vi "Autonomous.vi"   [LabVIEW 2017]
doc: "This VI starts when autonomous period begins, and will automatically be terminated when it ends. You can carry out timed or sensor driven operations directly to I/O or to subsystems without needing to return to the caller."
uses:
  <vilib>/Rock Robotics/WPI/Utilities/WPI_GetSetVariantRefNum.vi
  <vilib>/Rock Robotics/Network Tables/NT Read String.vi
types:
  T1 = typedef "Command Status Info.ctl" = cluster{"Name":string, "Status":T2, "notifier out":T3}
  T2 = typedef "Completion Status.ctl" = enum16{"Successful", "Aborted", "Incomplete"}
  T3 = typedef "Completion Notifier.ctl" = refnum<notifier>
  T4 = typedef "WPI_JoystickDevRef.ctl" = cluster{"Device":T5}
  T5 = typedef "WPI_JoystickDeviceEnum.ctl" = enum16{"USB 0", "USB 1", "USB 2", "USB 3", "USB 4", "USB 5"}
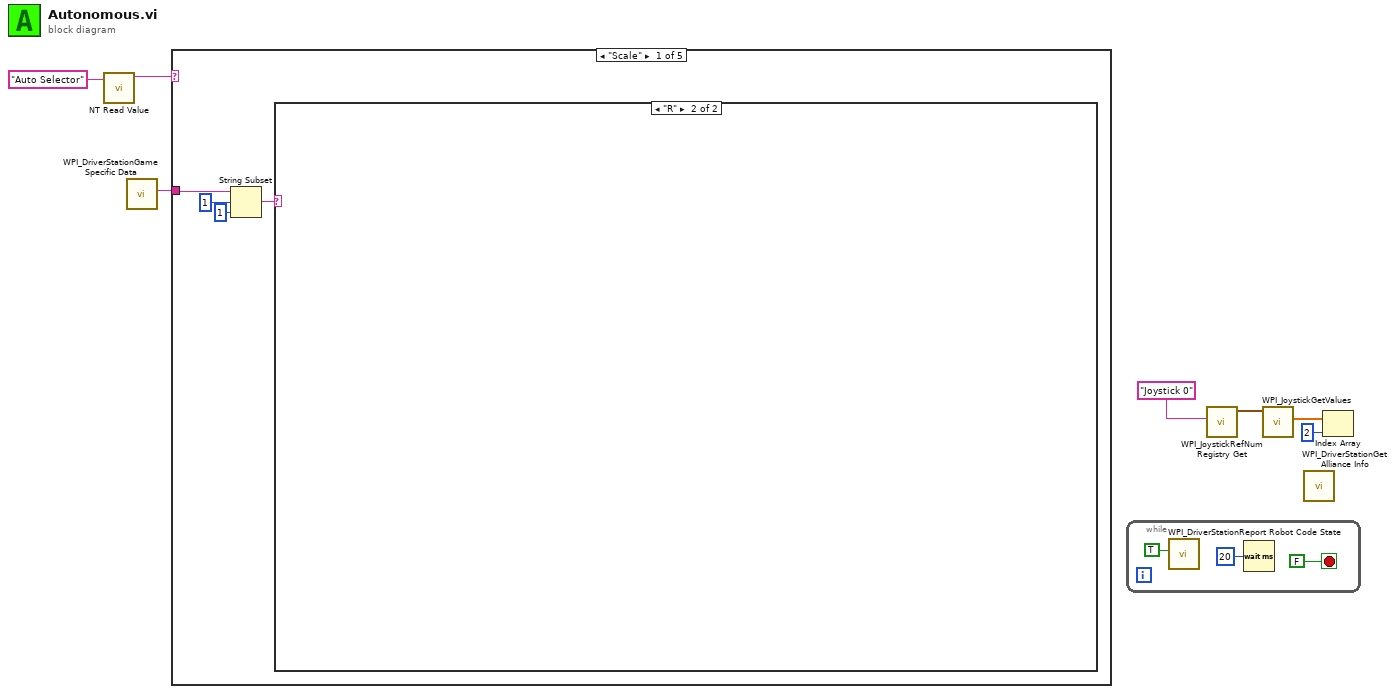
[diagram p0: block diagram]
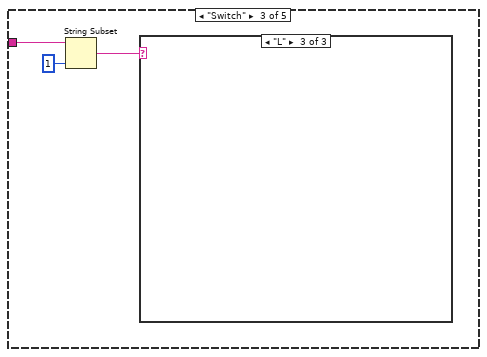
[diagram p4: hidden frame]
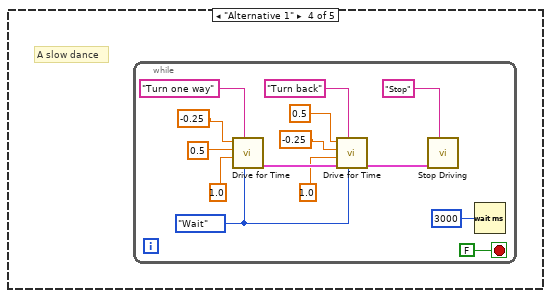
[diagram p7: hidden frame]
diagram:
  n1 = call-poly <vilib>:"NT Read Value.vi"("Name"="Auto Selector") -> ("String"=w2:string)  [unwired: 9 in, 1 out]
  n2 = call <vilib>:"WPI_DriverStationGame Specific Data.vi"() -> ("Game Specific Data"=w1:string)  [unwired: 11 in]
  n3 = case shown="\"Scale\"" w2 {
    tunnel: w1 -> [w11 _ w14 _ _]
    frame "Scale" {
      n4 = String Subset(string=w11, offset (0)=1, length (rest)=1 ("length (rest)")) -> (substring=w8:string)
      n5 = case shown="\"R\"" w8 {
        frame "L", Default {
        }
        frame "R" {
        }
      }
    }
    frame "Baseline" {
    }
    frame "Switch" {
      n6 = String Subset(string=w14, length (rest)=1 ("length (rest)")) -> (substring=w13:string)  [unwired: 1 in]
      n7 = case shown="\"L\"" w13 {
        frame "Def", Default {
        }
        frame "R" {
        }
        frame "L" {
        }
      }
    }
    frame "Alternative 1" {
      # "A slow dance"
      n8 = while {
        stop <- FALSE stop-if-true
        w19 = enum16{"Start", "Wait"}."Wait" ("Synchronication")
        n9 = call "Drive for Time.vi"("Synchronization"=w19, "Description"="Turn one way", "Seconds"=1.0 ("Delay (s)"), "Right Speed"=0.5 ("X axis value"), "Left Speed"=-0.25 ("X axis value")) -> ("Command Info Out"=w28:T1)  [unwired: 5 in, 1 out]
        n10 = call "Drive for Time.vi"("Synchronization"=w19, "Description"="Turn back", "Command Info In"=w28, "Seconds"=1.0 ("Delay (s)"), "Right Speed"=-0.25 ("X axis value"), "Left Speed"=0.5 ("X axis value")) -> ("Command Info Out"=w18:T1)  [unwired: 4 in, 1 out]
        n11 = call "Stop Driving.vi"("Description"="Stop", "Command Info In"=w18) -> ()  [unwired: 9 in, 1 out]
        n12 = Wait (ms)(milliseconds to wait=u32 3000 ("millisecond timer value")) -> ()  [unwired: 1 out]
      }
    }
    frame "Nothing", Default {
    }
  }
  n13 = while {
    stop <- FALSE stop-if-true
    n14 = call <vilib>:"WPI_DriverStationReport Robot Code State.vi"("Autonomous"=TRUE) -> ()  [unwired: 10 in, 1 out]
    n15 = Wait (ms)(milliseconds to wait=u32 20) -> ()  [unwired: 1 out]
  }
  n16 = call <vilib>:"WPI_JoystickRefNum Registry Get.vi"("refnum name"="Joystick 0") -> ("JoystickDevRef"=w6:T4)  [unwired: 1 in, 9 out]
  n17 = call <vilib>:"WPI_JoystickGetValues.vi"("JoystickDevRef"=w6) -> ("Axes"=w5:dbl[])  [unwired: 6 in, 4 out]
  n18 = call <vilib>:"WPI_DriverStationGet Alliance Info.vi"() -> ()  [unwired: 12 out]
  n19 = Index Array(array=w5, index=2) -> ()  [unwired: 1 out]
